vi "Sets the test number for MANU.vi"(5 "Enable to Query":bool, 7 "Enable to Setup":bool, 8 "error in":errorcluster, 10 "Test number":u8 max=100, 11 "VISA resource name":refnum<visa-resource-name>) -> (0 "error out":errorcluster, 2 "Return the Test number":string, 3 "VISA resource name out":refnum<visa-resource-name>)   [LabVIEW 2021, in "GPT-9000.lvlib"]
uses:
  GPT-9000.lvlib
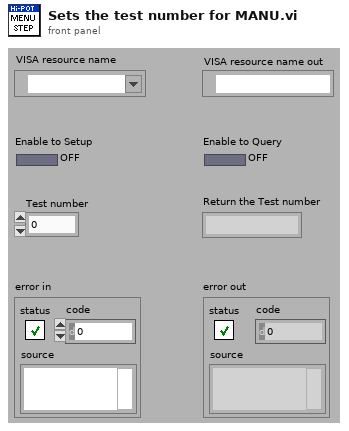
[diagram p1: front panel]
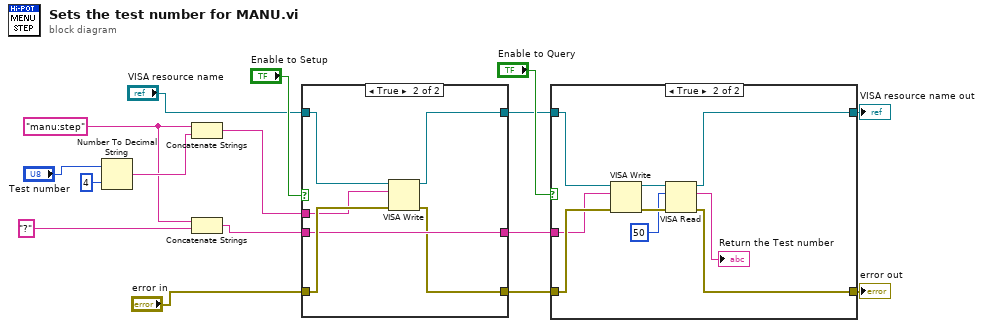
[diagram p0: block diagram]
diagram:
  w12 = "manu:step"
  n1 = Number To Decimal String(number="Test number", width (-)=i16 4) -> (decimal integer string=w14:string)
  n2 = Concatenate Strings(w12, w14) -> (w10:string)
  n3 = Concatenate Strings(w12, "?") -> (w9:string)
  n4 = case shown="True" "Enable to Setup" {
    tunnel: w10 -> [_ w23]
    tunnel: w9 -> [w17 w22]
    tunnel: "VISA resource name" -> [w19 w25]
    tunnel: "error in" -> [w18 w24]
    tunnel: [w19 w21] -> w5
    tunnel: [w18 w20] -> w4
    tunnel: [w17 w22] -> w1
    frame False {
    }
    frame True {
      n5 = VISA Write(VISA resource name=w25, write buffer=w23, error in (no error)=w24) -> (VISA resource name out=w21:refnum<visa-resource-name>, error out=w20:errorcluster)  [unwired: 1 out]
    }
  }
  n6 = case shown="True" "Enable to Query" {
    tunnel: w5 -> [w27 w36]
    tunnel: w4 -> [w26 w35]
    tunnel: [w27 w30] -> w3
    tunnel: [w26 w28] -> w2
    tunnel: w1 -> [_ w34]
    frame False {
    }
    frame True {
      n7 = VISA Write(VISA resource name=w36, write buffer=w34, error in (no error)=w35) -> (VISA resource name out=w33:refnum<visa-resource-name>, error out=w32:errorcluster)  [unwired: 1 out]
      n8 = VISA Read(VISA resource name=w33, byte count=u32 50, error in (no error)=w32) -> (VISA resource name out=w30:refnum<visa-resource-name>, read buffer=→"Return the Test number":string, error out=w28:errorcluster)  [unwired: 1 out]
    }
  }
  "VISA resource name out" <- w3
  "error out" <- w2
